vi "U8ArrayToI16.vi"(11 "U8 DATA IN":u8[](array[numeric])) -> (3 "I16 OUT":i16[](array[numeric]))   [LabVIEW 2017]
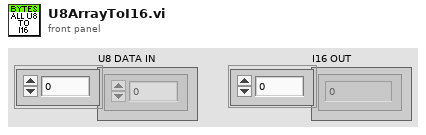
[diagram p1: front panel]
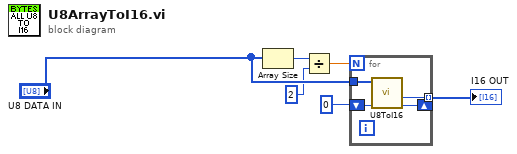
[diagram p0: block diagram]
diagram:
  n1 = Array Size(array="U8 DATA IN") -> (size(s)=w1:i32)
  n2 = Divide(x=w1, y=2 ("index")) -> (x/y=w3:dbl)
  n3 = for {
    N: w3 -> [_]
    tunnel: "U8 DATA IN" -> [w10]
    shift-right: [w8] -> _
    shift-left: 0 ("index") -> [w9]
    tunnel: [w7] -> w5 mode=indexing
    n4 = call "U8ToI16.vi"("Index"=w9, "Input U8 Array"=w10) -> ("Index+2"=w8:u32, "Output I16"=w7:i16)  [unwired: 3 in, 1 out]
  }
  "I16 OUT" <- w5
